vi "Cleanup.vi"(8 "error in (no error)":errorcluster, 11 "Scorer in":refnum<class "Scorer.lvclass">) -> (0 "error out":errorcluster)   [LabVIEW 2020, in "Summer of LabVIEW.lvlib" / "Scorer.lvclass"]
uses:
  Scorer.lvclass
  Scorer.lvclass/Scorer.ctl
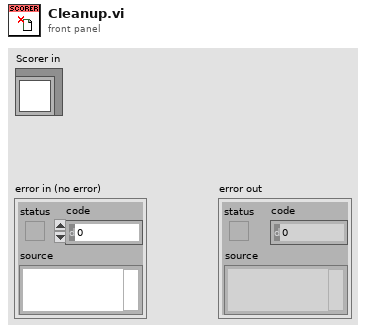
[diagram p1: front panel]
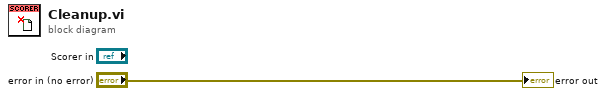
[diagram p0: block diagram]
diagram:
  "error out" <- "error in (no error)"
